vi "read-index.vi"(7 "dvr":refnum<data-value>, 8 "error in (no error)":errorcluster) -> (0 "error out":errorcluster, 3 "index":i32)   [LabVIEW 2015, in "lv-graph-global.lvlib"]
doc: "read_index can be used to read the current index of the data in the DVR."
uses:
  _controls/data.ctl
  _controls/configuration.ctl
  _controls/store_method.ctl
  lv-graph-global.lvlib
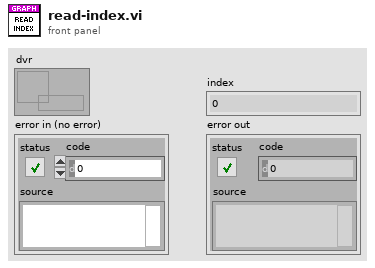
[diagram p1: front panel]
types:
  T1 = typedef "lv-graph-global.lvlib/data.ctl" = cluster{"configuration":T2, "index":i32, "x_axis":dbl[], "y_axis":dbl[][]}
  T2 = typedef "lv-graph-global.lvlib/configuration.ctl" = cluster{"store_method":T3, "rows":i32, "columns":i32}
  T3 = typedef "lv-graph-global.lvlib/store_method.ctl" = enum16{"<store_method>", "fixed", "grow"}
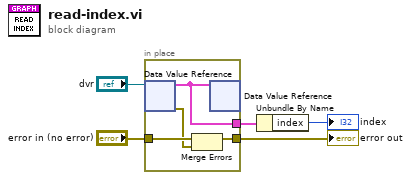
[diagram p0: block diagram]
diagram:
  n1 = in-place {
    in-place-border: [w9] -> w4
    in-place-border: "error in (no error)" -> [w8]
    in-place-border: [w6] -> w2
    n2 = in-place-dvr #1("dvr") -> (w9:T1, w7:errorcluster)
    n3 = Merge Errors(w8, w7) -> (w6:errorcluster)
    n4 = in-place-dvr #1(w9) -> ()  [unwired: 2 out]
  }
  "error out" <- w2
  n5 = Unbundle By Name(w4) -> ("index"=→"index":i32)
